vi "WT300 Create List.vi"(8 "error in (no error)":errorcluster, 10 "Element (1: 1)":i32, 11 "VISA Refnum in":refnum<visa-resource-name>) -> (0 "error out":errorcluster, 1 "UTDH Index":i32, 2 "Number of Items":i32, 3 "VISA Refnum out":refnum<visa-resource-name>)   [LabVIEW 2019]
uses:
  Public/Utility/Function/Create Function String (Frequency).vi
  Public/Utility/Function/Create Function String (Power).vi
  Public/Utility/Function/Create Function String (Current).vi
  Public/Utility/Function/Create Function String (Voltage).vi
  Public/Utility/Function/Create Function String (Harmonics).vi
  Public/Utility/Function/Create Function String (Integrate).vi
  Yokogawa WT300 Series.lvlib
panel:
  out "appended array":string[](array[string])
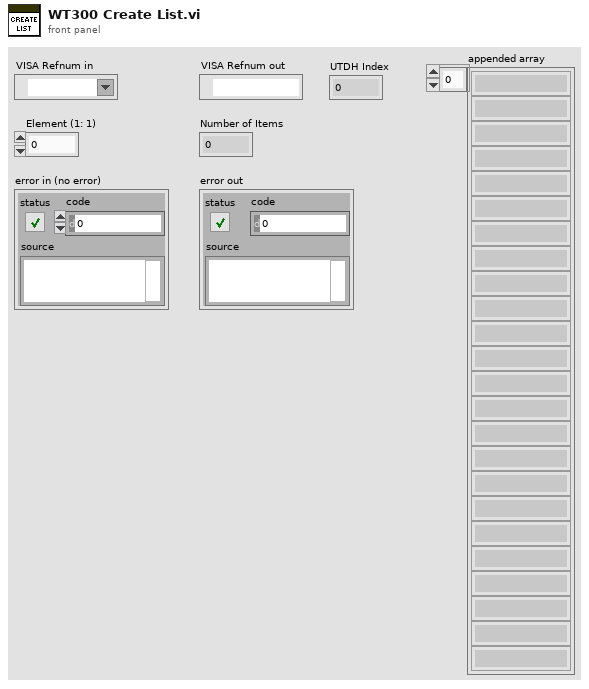
[diagram p1: front panel]
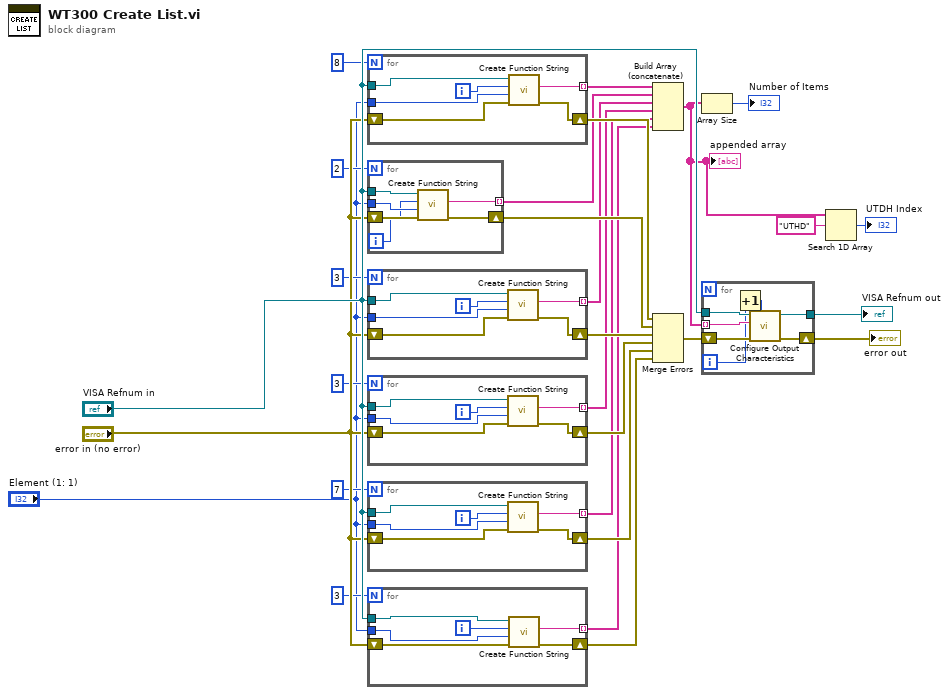
[diagram p0: block diagram]
diagram:
  n1 = for {
    N: 8 -> [_]
    tunnel: "VISA Refnum in" -> [w34]
    tunnel: [w33] -> w6 mode=indexing
    tunnel: "Element (1: 1)" -> [w32]
    shift-right: [w29] -> w18
    shift-left: "error in (no error)" -> [w30]
    i -> [w31]
    n2 = call-poly "Create Function String.vi"("error in (no error)"=w30, "Element (1: 1)"=w32, "Function (0: Time)"=w31, "VISA resource name"=w34) -> ("error out"=w29:errorcluster, "Function String"=w33:string)  [unwired: 5 in, 1 out]
  }
  n3 = for {
    N: 2 -> [_]
    tunnel: [w40] -> w4 mode=indexing
    tunnel: "VISA Refnum in" -> [w39]
    tunnel: "Element (1: 1)" -> [w38]
    shift-right: [w36] -> w19
    shift-left: "error in (no error)" -> [w37]
    i -> [w35]
    n4 = call-poly "Create Function String.vi"("error in (no error)"=w37, "Element (1: 1)"=w38, "Function (0: Uthd)"=w35, "VISA resource name"=w39) -> ("error out"=w36:errorcluster, "Function String"=w40:string)  [unwired: 5 in, 1 out]
  }
  n5 = for {
    N: 3 -> [_]
    tunnel: "VISA Refnum in" -> [w46]
    tunnel: [w45] -> w7 mode=indexing
    tunnel: "Element (1: 1)" -> [w44]
    shift-right: [w41] -> w20
    shift-left: "error in (no error)" -> [w42]
    i -> [w43]
    n6 = call-poly "Create Function String.vi"("error in (no error)"=w42, "Element (1: 1)"=w44, "Function (0: U)"=w43, "VISA resource name"=w46) -> ("error out"=w41:errorcluster, "Function String"=w45:string)  [unwired: 5 in, 1 out]
  }
  n7 = for {
    N: 3 -> [_]
    tunnel: "VISA Refnum in" -> [w52]
    tunnel: [w51] -> w8 mode=indexing
    tunnel: "Element (1: 1)" -> [w50]
    shift-right: [w47] -> w21
    shift-left: "error in (no error)" -> [w48]
    i -> [w49]
    n8 = call-poly "Create Function String.vi"("error in (no error)"=w48, "Element (1: 1)"=w50, "Function (0: I)"=w49, "VISA resource name"=w52) -> ("error out"=w47:errorcluster, "Function String"=w51:string)  [unwired: 5 in, 1 out]
  }
  n9 = for {
    N: 7 -> [_]
    tunnel: "VISA Refnum in" -> [w58]
    tunnel: [w57] -> w9 mode=indexing
    tunnel: "Element (1: 1)" -> [w56]
    shift-right: [w53] -> w22
    shift-left: "error in (no error)" -> [w54]
    i -> [w55]
    n10 = call-poly "Create Function String.vi"("error in (no error)"=w54, "Element (1: 1)"=w56, "Function (0: P)"=w55, "VISA resource name"=w58) -> ("error out"=w53:errorcluster, "Function String"=w57:string)  [unwired: 5 in, 1 out]
  }
  n11 = for {
    N: 3 -> [_]
    tunnel: "VISA Refnum in" -> [w64]
    tunnel: [w63] -> w10 mode=indexing
    tunnel: "Element (1: 1)" -> [w62]
    shift-right: [w59] -> w23
    shift-left: "error in (no error)" -> [w60]
    i -> [w61]
    n12 = call-poly "Create Function String.vi"("error in (no error)"=w60, "Element (1: 1)"=w62, "Function (0: Frequency U)"=w61, "VISA resource name"=w64) -> ("error out"=w59:errorcluster, "Function String"=w63:string)  [unwired: 5 in, 1 out]
  }
  n13 = Build Array (concatenate)(w6, w4, w7, w8, w9, w10) -> (w3:string[])
  "appended array" <- w3
  n14 = Merge Errors(w18, w19, w20, w21, w22, w23) -> (w24:errorcluster)
  n15 = Array Size(array=w3) -> (size(s)=→"Number of Items":i32)
  n16 = for {
    tunnel: w3 -> [w71] mode=indexing
    tunnel: "VISA Refnum in" -> [w70]
    tunnel: [w69] -> w26
    shift-right: [w68] -> w25
    shift-left: w24 -> [w67]
    i -> [w66]
    n17 = Increment(x=w66) -> (x+1=w65:i32)
    n18 = call "Configure Output Characteristics.vi"("Item (1)"=w65, "error in (no error)"=w67, "Function (Empty)"=w71, "VISA resource name"=w70) -> ("error out"=w68:errorcluster, "VISA resource name out"=w69:refnum<visa-resource-name>)  [unwired: 6 in]
  }
  "VISA Refnum out" <- w26
  "error out" <- w25
  n19 = Search 1D Array(1D array=w3, element="UTHD") -> (index of element=→"UTDH Index":i32)  [unwired: 1 in]
